vi "passTestBallTouchesRobot.vi"(6 "Thread organizer":T2, 9 "Kicker robot":T1, 10 "IA State":T3) -> (2 "Receveing Robot":T1)   [LabVIEW 2017]
uses:
  <extravilib>/ChannelInstances/Lossy Stream-t'AI Input.ctl'/)Channel.ctl
  Core/AI Input.ctl
  Core/AI Robot.ctl
  Intel/Functions Enum.ctl
  Intel/AttackerStates.ctl
  Core/AI Ball.ctl
  Core/Field Size.ctl
  Core/AI Judge.ctl
  Intel/Command Enum.ctl
  Util/Events/Events.ctl
  <extravilib>/ChannelInstances/Lossy Stream-dbl/)Channel.ctl
  <extravilib>/ChannelInstances/Lossy Stream-t'passTestStates.ctl'/)Channel.ctl
  passTestStates.ctl
  <extravilib>/ChannelInstances/Lossy Stream-t'passTestStates.ctl'/Read With Abort.vi
  <extravilib>/ChannelInstances/Lossy Stream-dbl/Read With Abort.vi
  <extravilib>/ChannelInstances/Lossy Stream-t'AI Input.ctl'/Read With Abort.vi
  <extravilib>/ChannelInstances/Lossy Stream-dbl/Write With Abort.vi
  <extravilib>/ChannelInstances/Lossy Stream-t'passTestStates.ctl'/EndpointRead.vi
  <extravilib>/ChannelInstances/Lossy Stream-dbl/EndpointRead.vi
  <extravilib>/ChannelInstances/Lossy Stream-t'AI Input.ctl'/EndpointRead.vi
  <extravilib>/ChannelInstances/Lossy Stream-dbl/Endpoint.vi
  <extravilib>/ChannelInstances/Lossy Stream-t'passTestStates.ctl'/)Channel.vi
  <resource>/ChannelSupport/_ChannelSupport/WaitIfNeeded.vi
  <extravilib>/ChannelInstances/Lossy Stream-dbl/)Channel.vi
  <extravilib>/ChannelInstances/Lossy Stream-t'AI Input.ctl'/)Channel.vi
  <extravilib>/ChannelInstances/Lossy Stream-t'AI Input.ctl'.lvlib
  <extravilib>/ChannelInstances/Lossy Stream-dbl.lvlib
  <extravilib>/ChannelInstances/Lossy Stream-t'passTestStates.ctl'.lvlib
panel:
  out "Receveing robot":dbl
  out "Comm FPS 7":dbl
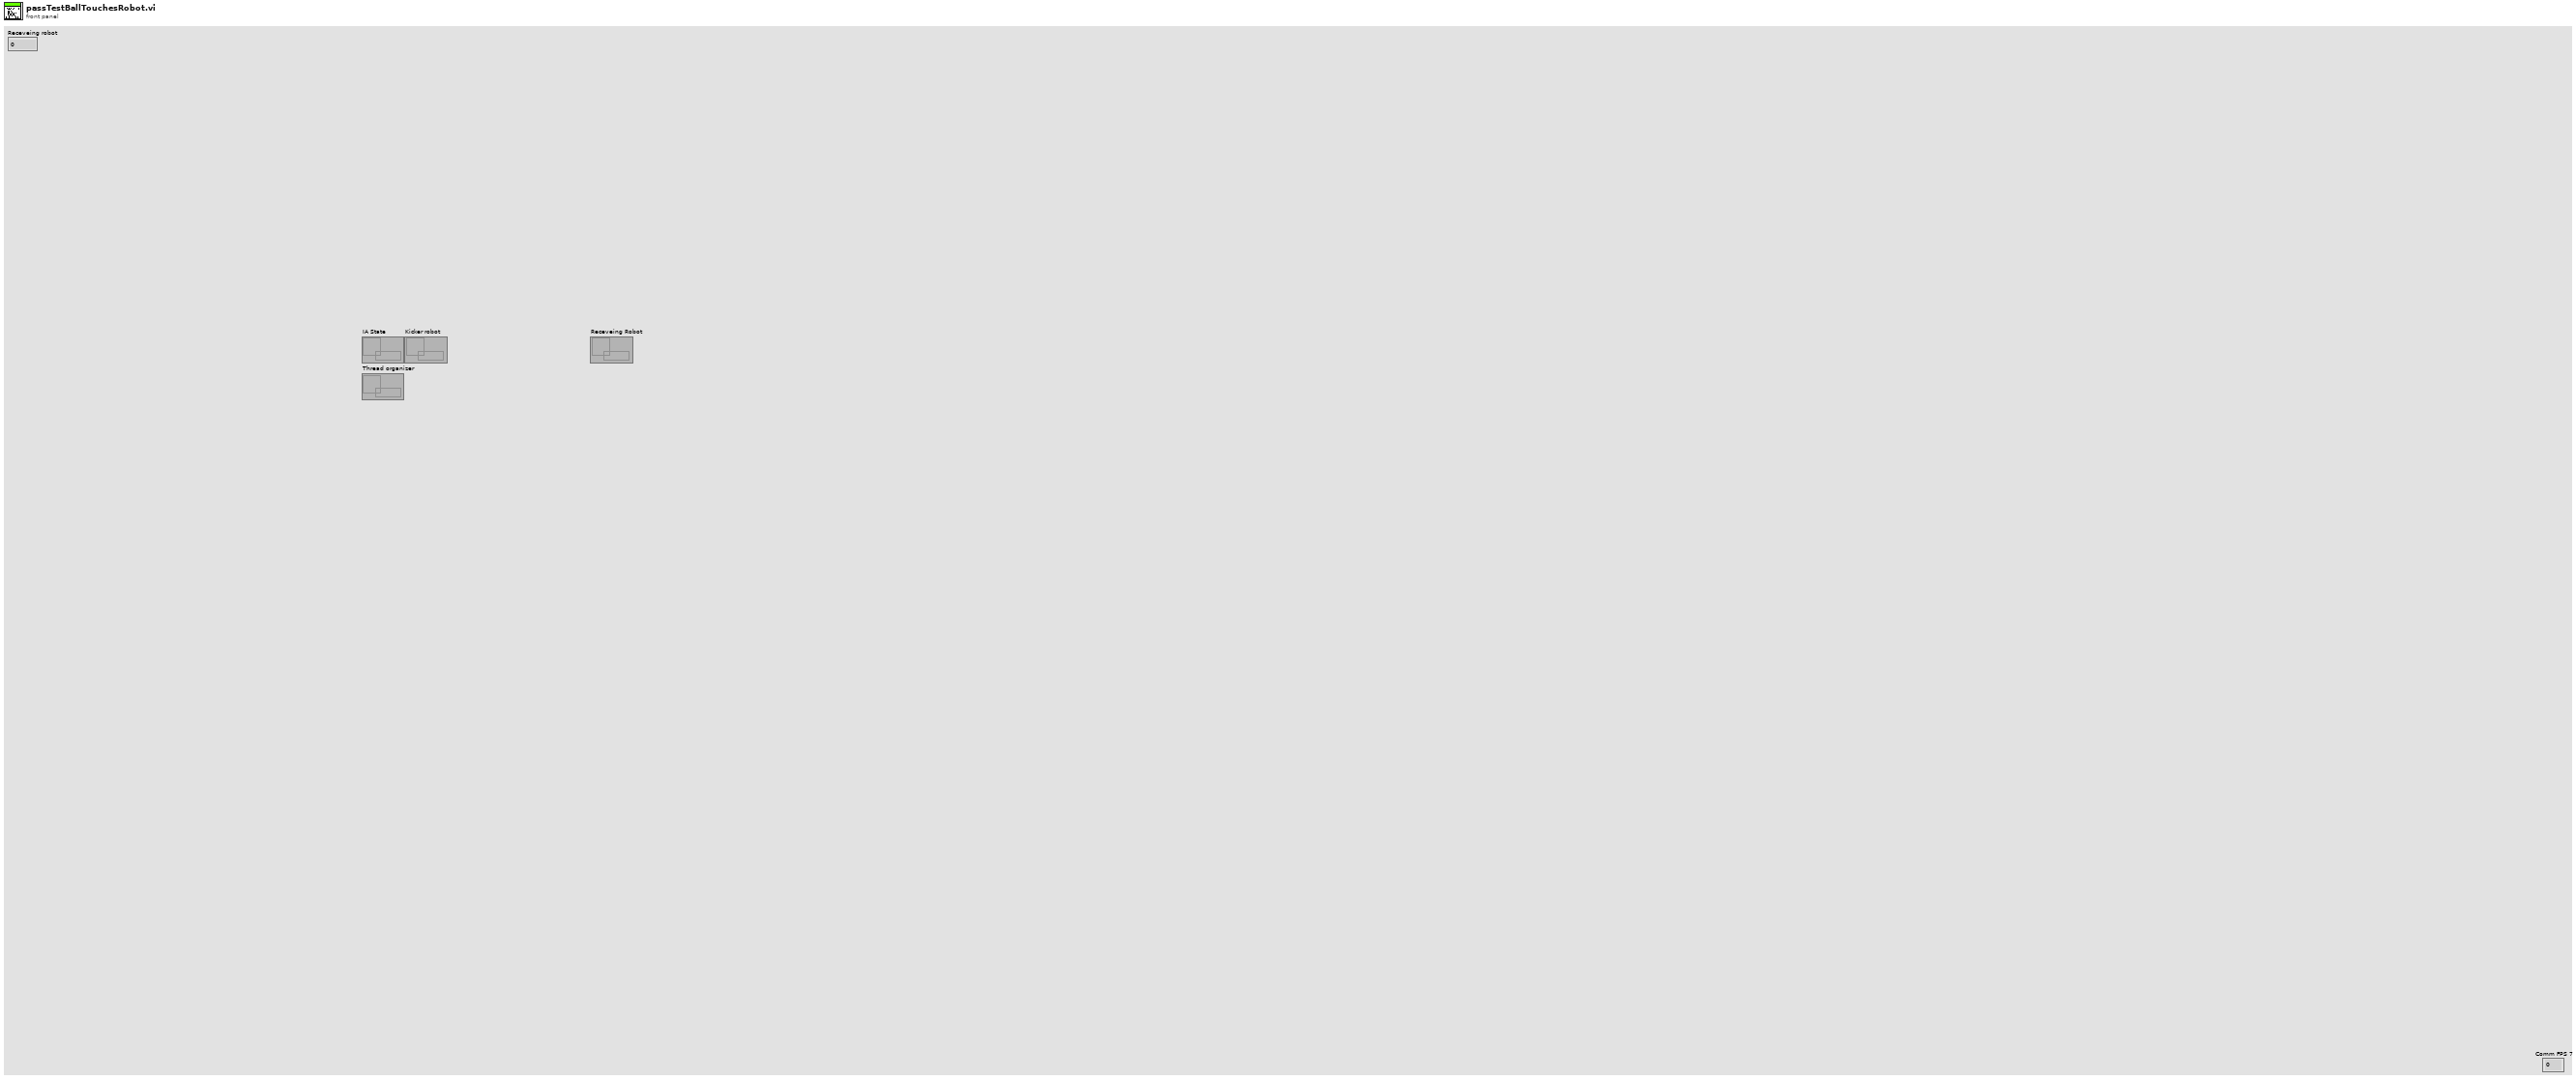
[diagram p1: front panel]
types:
  T1 = typedef "Lossy Stream-dbl.lvlib/)Channel.ctl" = refnum<queue>
  T2 = typedef "Lossy Stream-t'passTestStates.ctl'.lvlib/)Channel.ctl" = refnum<queue>
  T3 = typedef "Lossy Stream-t'AI Input.ctl'.lvlib/)Channel.ctl" = refnum<queue>
  T4 = typedef "passTestStates.ctl" = enum16{"Pass on the way", "Ball stops", "Pass intercepted", "Ball out of the field", "Ball missed robot", "Need more force to pass", "Too much force", "Correct pass", "Keep ball possesion", "Robot kicked the ball", "Waiting Kick", "Invalid: same robot", "Invalid: kicker ID 999", "Invalid: Receiver ID 999", "Invalid"}
  T5 = typedef "AI Input.ctl" = cluster{"our_robots":T6[], "enemy_robots":T6[], "balls":T9[], "geometry":T10, "IA Judge":T11, "Received Timestamp":timestamp, "Events":T13}
  T6 = typedef "AI Robot.ctl" = cluster{"id":u32, "function":T7, "x":dbl, "y":dbl, "orientation":dbl, "v_tangent":dbl, "v_normal":dbl, "v_ang":dbl, "kick_x":dbl, "kick_z":dbl, "dribble":bool, "Timestamp":timestamp, "dest_x":dbl, "dest_y":dbl, "dest_orientation":dbl, "estimatives":cluster{"est_v_tangent":dbl, "est_v_normal":dbl, "est_vx":dbl, "est_vy":dbl, "Pos Robot Est":dbl[]}, "dest_x_kick":dbl, "dest_y_kick":dbl, "Gap Coord":dbl[], "States":T8}
  T7 = typedef "Functions Enum.ctl" = enum16{"Attacker", "Goalie", "Defender", "Striker", "Goto 0", "Dummy", "Kicker", "ZigZag"}
  T8 = typedef "AttackerStates.ctl" = enum16{"Pass", "GoToTangent", "BallGetting", "GoToKick", ""}
  T9 = typedef "AI Ball.ctl" = cluster{"x":dbl, "y":dbl, "timestamp":timestamp, "Vel_x":dbl, "Vel_y":dbl, "Pos Bola Est":dbl[]}
  T10 = typedef "Field Size.ctl" = cluster{"line_width":u32, "field_length":u32, "field_width":u32, "boundary_width":u32, "referee_width":u32, "goal_width":u32, "goal_depth":u32, "goal_wall_width":u32, "center_circle_radius":u32, "defense_radius":u32, "defense_stretch":u32, "free_kick_from_defense_dist":u32, "penalty_spot_from_field_line_dist":u32, "penalty_line_from_spot_dist":u32}
  T11 = typedef "AI Judge.ctl" = cluster{"stage":string, "command":string, "our_goalie_id":dbl, "enemy_goalie_id":dbl, "command enum":T12, "Time":enum16{"Azul", "Amarelo"}}
  T12 = typedef "Command Enum.ctl" = enum16{"Halt", "Stop", "Force Start", "PKA Normal Start", "Prepare Kickoff Ally", "PKE Normal Start", "Prepare Kickoff Enemy", "Prepare Penalty Ally", "PPA Normal Start", "Prepare Penalty Enemy", "PPE Normal Start", "Direct Free Enemy", "Direct Free Ally", "Indirect Free Enemy", "Indirect Free Ally", "Timeout Enemy", "Timeout Ally", "Goal Enemy", "Goal Ally", "Ball Placement Enemy", "Ball Placement Ally", "Normal Half Time", "Extra Time Break", "Extra Half Time", "None", "Post Game"}
  T13 = typedef "Events.ctl" = cluster{"Touch":bool, "Ball out":bool, "id touch":dbl, "Ball out of \nVision":bool, "Ball inside \nGoalie area":bool, "Robot not responding":bool, "Robots responding status":dbl[], "Enemy Ball \nPossession":bool, "Pass State":bool, "id end of pass":dbl, "Kick":bool, "Id ini Possession":dbl, "Ball Possesion":bool, "Id Possesion":dbl}
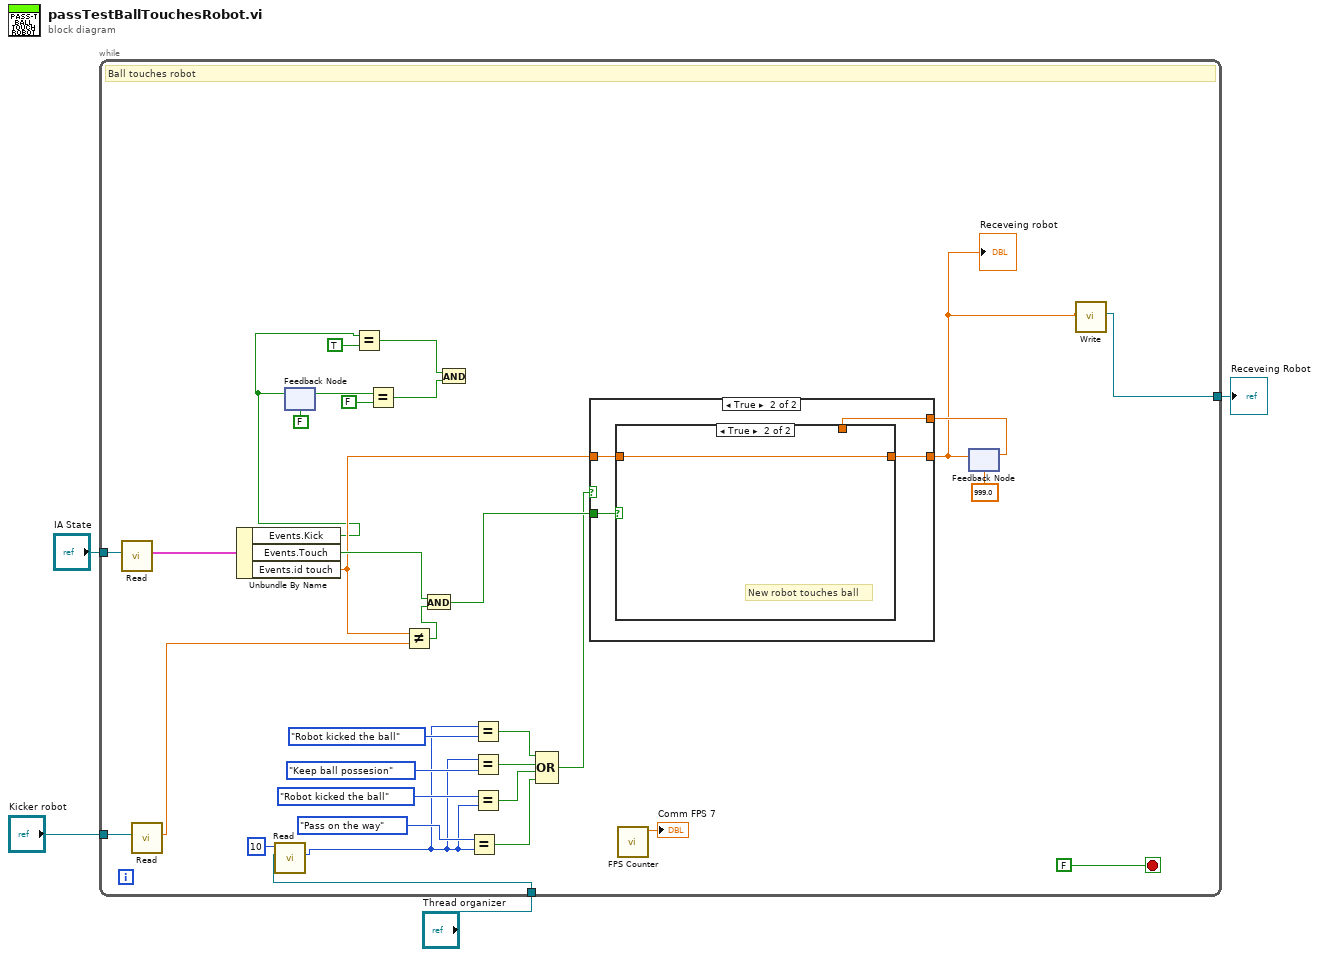
[diagram p0: block diagram]
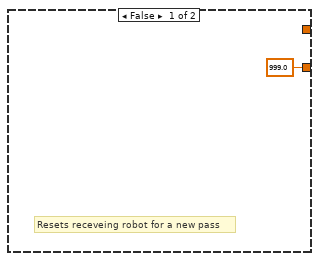
[diagram p2: hidden frame]
diagram:
  n1 = while {
    tunnel: "IA State" -> [w36]
    tunnel: "Kicker robot" -> [w34]
    tunnel: [w27] -> w1
    tunnel: "Thread organizer" -> [w17]
    stop <- FALSE stop-if-true
    # "Ball touches robot"
    n2 = call <extravilib>:"Read.vi"("channel"=w36) -> ("element"=w26:T5)  [unwired: 5 in, 5 out]
    n3 = call <extravilib>:"Read.vi"("channel"=w34) -> ("element"=w33:dbl)  [unwired: 5 in, 5 out]
    n4 = Unbundle By Name(w26) -> ("Events.Kick"=w19:bool, "Events.Touch"=w32:bool, "Events.id touch"=w29:dbl)
    n5 = call <extravilib>:"Read.vi"("channel"=w17, "timeout in ms (-1)"=10) -> ("element"=w12:T4)  [unwired: 4 in, 5 out]
    n6 = feedback #1(FALSE ("Kick")) -> (w23:bool)
    n7 = feedback-in #1(w19) -> ()
    n8 = Equal?(x=w19, y=TRUE) -> (x = y?=w20:bool)
    n9 = Equal?(x=w23, y=FALSE) -> (x = y?=w21:bool)
    n10 = Not Equal?(x=w29, y=w33) -> (x != y?=w31:bool)
    n11 = And(x=w32, y=w31) -> (x .and. y?=w30:bool)
    n12 = And(x=w20, y=w21) -> ()  [unwired: 1 out]
    n13 = Equal?(x=passTestStates."Pass on the way" ("y"), y=w12) -> (x = y?=w11:bool)
    n14 = Equal?(x=w12, y=passTestStates."Robot kicked the ball") -> (x = y?=w8:bool)
    n15 = Equal?(x=w12, y=passTestStates."Keep ball possesion") -> (x = y?=w9:bool)
    n16 = Equal?(x=passTestStates."Robot kicked the ball" ("y"), y=w12) -> (x = y?=w10:bool)
    n17 = Compound Arithmetic op=OR(w8, w9, w10, w11) -> (w7:bool)
    n18 = call "FPS Counter.vi"() -> ("Numeric"=→"Comm FPS 7":dbl)  [unwired: 11 in]
    n19 = feedback #2(999.0 ("id touch")) -> (w28:dbl)
    n20 = case shown="True" w7 {
      tunnel: w30 -> [_ w42]
      tunnel: w29 -> [_ w41]
      tunnel: w28 -> [_ w40]
      tunnel: [999.0 ("id touch") w39] -> w18
      frame False {
        # "Resets receveing robot for a new pass"
      }
      frame True {
        n21 = case shown="True" w42 {
          tunnel: w41 -> [_ w44]
          tunnel: [w43 w44] -> w39
          tunnel: w40 -> [w43 _]
          frame False {
          }
          frame True {
            # "New robot touches ball"
          }
        }
      }
    }
    "Receveing robot" <- w18
    n22 = feedback-in #2(w18) -> ()
    n23 = call <extravilib>:"Write.vi"("element"=w18) -> ("channel"=w27:T1)  [unwired: 8 in, 2 out]
  }
  "Receveing Robot" <- w1
